vi "LEO PROVA MINCHIATA 2 RT.vi"() -> ()   [LabVIEW 2014]
uses:
  <vilib>/FPGAPlugInAG/sbRIO-9636/niLvFpga_Open_sbRIO-9636.vi
  <vilib>/rvi/interface/common/dynamic/niFpgaDynamicAddResources.vi
  <vilib>/Utility/error.llb/Error Cluster From Error Code.vi
  <vilib>/rvi/errors/niLvFpgaAdjustHostInterfaceError.vi
  <vilib>/rvi/interface/common/niFpgaWaitOnOcc.vi
  <vilib>/FPGAPlugInAG/Dynamic/niLvFpga_Run_Dynamic.vi
  <vilib>/FPGAPlugInAG/Dynamic/niLvFpga_Abort_Dynamic.vi
  <vilib>/FPGAPlugInAG/Dynamic/niLvFpga_Close_Dynamic.vi
  <vilib>/rvi/interface/nirviOpenFPGA/nirviOpenFPGA.xnode
  FPGA Bitfiles/LaserDistanceSen_FPGATarget_LEOPROVAMINCHIAT_fFqByPhw9ZU.lvbitx
  FPGA Target/Test VIs/LEO PROVA MINCHIATA 2.vi
  <vilib>/rvi/interface/nirviReadWriteControl/nirviReadWriteControl.xnode
  <vilib>/rvi/interface/nirviMethod/nirviMethod.xnode
  <vilib>/rvi/interface/nirviCloseFPGA/nirviCloseFPGA.xnode
  <vilib>/FPGAPlugInAG/Dynamic/niLvFpga_ConfigureFifo_Dynamic.vi
  <vilib>/rvi/errors/niLvFpgaMergeErrorWithErrorCode.vi
  <vilib>/FPGAPlugInAG/Dynamic/niLvFpga_StartFifo_Dynamic.vi
  <vilib>/rvi/interface/Simulation/niFpgaSimulationCallBeginRW.vi
  NiFpgaLv.dll
panel:
  in  "Windowing":T1(ring)
  in  "first bin":i32=10
  in  "last bin":i32=255
  in  "lower limit 2":u32(slide)=677 scale=625.0..737.0
  in  "lower limit 1":u32(slide)=59 scale=0.0..112.0
  out "Detected Frequency Tone - (Hz)":dbl
  in  "stop":bool
  out "Max Bin":i32
  out "Max Amp":dbl format="%.2f"
  out "Prev Bin":i32
  out "Next Bin":i32
  out "Prev Amp":dbl format="%.2f"
  out "Next Amp":dbl format="%.2f"
  out "Interpolated Bin":dbl
  in  "Interpolation Method":T2(ring)=enum."Jain"
  # "ONLINE parameter"
  # "OFFLINE parameters"
  # "Max Detection FFT bin range"
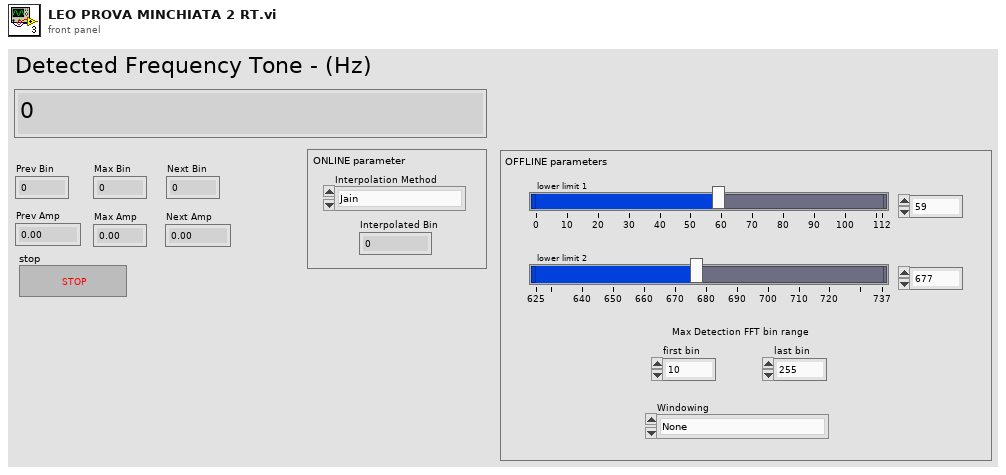
[diagram p1: front panel]
types:
  T1 = enum16{"None", "Hanning", "Hamming", "Blackman", "Blackman-Harris"}
  T2 = enum16{"Quadratic", "McLeodd", "Barycentric", "Jain"}
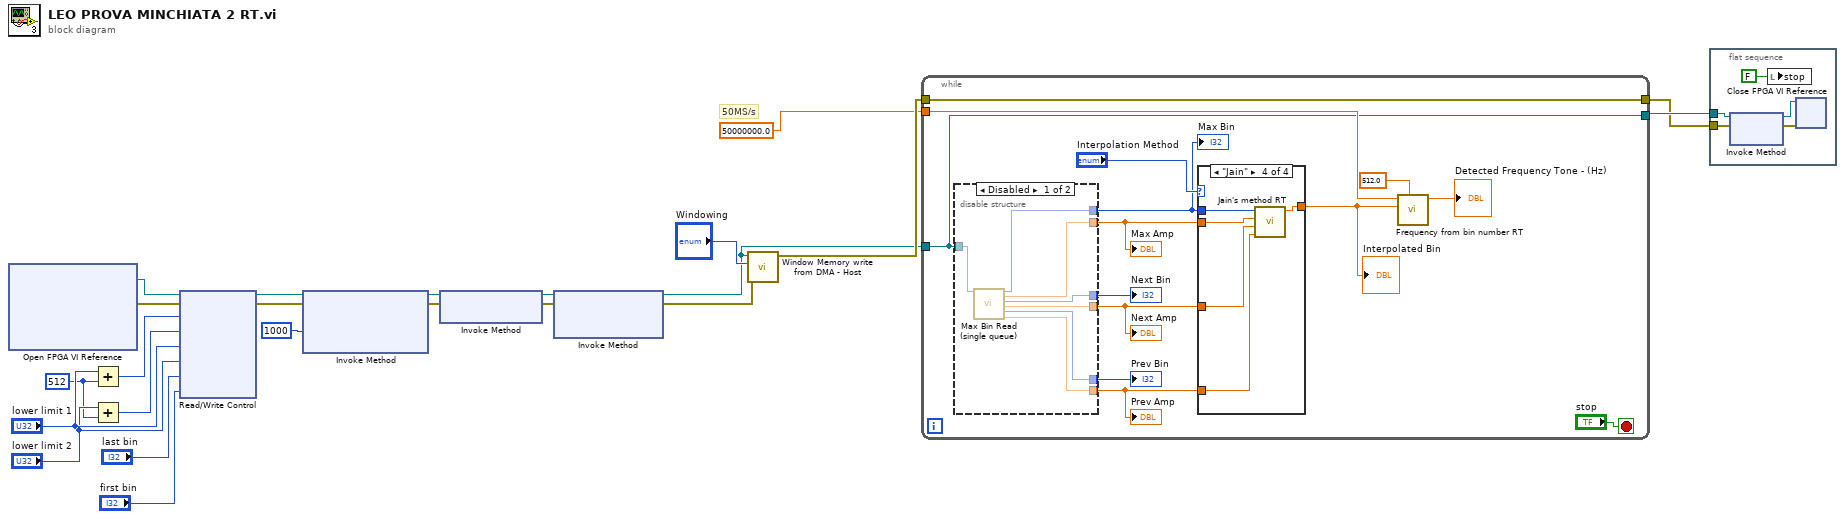
[diagram p0: block diagram]
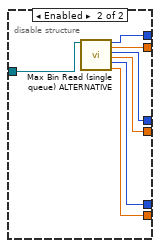
[diagram p2: hidden frame]
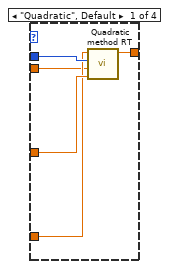
[diagram p3: hidden frame]
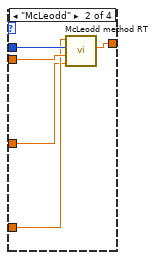
[diagram p4: hidden frame]
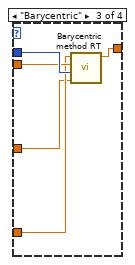
[diagram p5: hidden frame]
diagram:
  w17 = u32 512 ("y")
  # "50MS/s"
  n1 = xnode "Open FPGA VI Reference"() -> ("FPGA VI Reference Out"=w16:refnum<k20>, "error out"=w15:errorcluster)  [unwired: 2 in]
  n2 = Add(x="lower limit 1", y=w17) -> (x+y=w21:u32)
  n3 = Add(x="lower limit 2", y=w17) -> (x+y=w19:u32)
  n4 = xnode "Read/Write Control"("FPGA VI Reference In"=w16, "error in"=w15, "upper limit 1"=w21, "upper limit 2"=w19, "lower limit 1"="lower limit 1", "lower limit 2"="lower limit 2", "last bin"="last bin", "first bin"="first bin") -> ("FPGA VI Reference Out"=w9:refnum<k20>, "error out"=w8:errorcluster)
  n5 = xnode "Invoke Method"("FPGA VI Reference In"=w9, "error in"=w8, "Requested Depth"=u32 1000) -> ("FPGA VI Reference Out"=w7:refnum<k20>, "error out"=w6:errorcluster)  [unwired: 1 out]
  n6 = xnode "Invoke Method"("FPGA VI Reference In"=w7, "error in"=w6) -> ("FPGA VI Reference Out"=w4:refnum<k20>, "error out"=w5:errorcluster)
  n7 = xnode "Invoke Method"("FPGA VI Reference In"=w4, "error in"=w5) -> ("FPGA VI Reference Out"=w1:refnum<k20>, "error out"=w2:errorcluster)  [unwired: 1 in]
  n8 = call "Window Memory write from DMA - Host.vi"("error in"=w2, "Enum"="Windowing", "FPGA VI Reference In"=w1) -> ("error out"=w12:errorcluster)  [unwired: 5 in, 3 out]
  n9 = while {
    tunnel: 50000000.0 ("Sample Rate (S/s)") -> [w36]
    tunnel: w12 -> [w35]
    tunnel: [w24] -> w14
    tunnel: [w35] -> w3
    tunnel: w1 -> [w24]
    stop <- "stop" stop-if-true
    n10 = disable-structure shown="Disabled" {
      disable-tunnel: [w44 w51] -> w31
      disable-tunnel: [w43 w50] -> w30
      disable-tunnel: [w42 w48] -> w29
      disable-tunnel: [w41 w46] -> w28
      disable-tunnel: [w40 w47] -> w27
      disable-tunnel: [w39 w49] -> w26
      disable-tunnel: w24 -> [w38 w45]
      frame Disabled {
        n11 = call "Max Bin Read (single queue).vi"("FPGA VI Reference In"=w38) -> ("Max Bin"=w44:i32, "Max Amp"=w43:dbl, "Next Bin"=w39:i32, "Next Amp"=w42:dbl, "Prev Bin"=w40:i32, "Prev Amp"=w41:dbl)  [unwired: 13 in]
      }
      frame Enabled {
        n12 = call "Max Bin Read (single queue) ALTERNATIVE.vi"("FPGA VI Reference In"=w45) -> ("Max Bin"=w51:i32, "Max Amp"=w50:dbl, "Next Bin"=w49:i32, "Next Amp"=w48:dbl, "Prev Bin"=w47:i32, "Prev Amp"=w46:dbl)  [unwired: 13 in]
      }
    }
    "Max Bin" <- w31
    "Max Amp" <- w30
    "Prev Bin" <- w27
    "Next Bin" <- w26
    "Prev Amp" <- w28
    "Next Amp" <- w29
    n13 = case shown="\"Jain\"" "Interpolation Method" {
      tunnel: w31 -> [w55 w60 w65 w70]
      tunnel: w30 -> [w52 w59 w64 w69]
      tunnel: w28 -> [w53 w58 w63 w68]
      tunnel: w29 -> [w54 w57 w62 w67]
      tunnel: [w56 w61 w66 w71] -> w32
      frame "Quadratic", Default {
        n14 = call "Quadratic method RT.vi"("Next Amplitude"=w54, "Max Amplitude"=w52, "Max bin"=w55, "Prev Amplitude"=w53) -> ("Bin"=w56:dbl)  [unwired: 7 in]
      }
      frame "McLeodd" {
        n15 = call "McLeodd method RT.vi"("Next Amp"=w57, "Max Amp"=w59, "Max Bin"=w60, "Prev Amp"=w58) -> ("Bin"=w61:dbl)  [unwired: 7 in]
      }
      frame "Barycentric" {
        n16 = call "Barycentric method RT.vi"("Next Amp"=w62, "Max Bin"=w65, "Max Amp"=w64, "Prev Amp"=w63) -> ("Bin"=w66:dbl)  [unwired: 7 in]
      }
      frame "Jain" {
        n17 = call "Jain's method RT.vi"("Prev Amp"=w68, "Next Amp"=w67, "Max Amp"=w69, "Max Bin"=w70) -> ("Bin"=w71:dbl)  [unwired: 7 in]
      }
    }
    "Interpolated Bin" <- w32
    n18 = call "Frequency from bin number RT.vi"("FFT size"=512.0, "Bin number"=w32, "Sample Rate (S/s)"=w36) -> ("Detected Frequency (Hz)"=→"Detected Frequency Tone - (Hz)":dbl)  [unwired: 8 in]
  }
  n19 = flat-sequence {
    tunnel: w14 -> [w74]
    tunnel: w3 -> [w73]
    frame #0 {
      n20 = xnode "Invoke Method"("FPGA VI Reference In"=w74, "error in"=w73) -> ("FPGA VI Reference Out"=w75:refnum<k20>, "error out"=w76:errorcluster)
      n21 = local write "stop"(FALSE ("stop")) -> ()
      n22 = xnode "Close FPGA VI Reference"("FPGA VI Reference In"=w75, "error in"=w76) -> ()  [unwired: 1 out]
    }
  }
